vi "T7 Stream Error Handler KAG.vi"(8 "error in":errorcluster, 9 "Status Code":i32 format="%0.0f", 10 "Error Code":i32 format="%0.0f", 11 "Error Source":string) -> (0 "error out":errorcluster)   [LabVIEW 2022 SP3]
uses:
  <vilib>/Utility/error.llb/DialogType.ctl
panel:
  in  "Status Codes & Descriptions":cluster{"Codes":i32, "Descriptions":string}[](array[cluster])=[{"Codes"=2940, "Descriptions"="Auto-Recovery Active"}, {"Codes"=2941, "Descriptions"="Auto-Recovery End. Additional Status info = # scans skipped"}, {"Codes"=2942, "Descriptions"="Scan Overlap"}, {"Codes"=2943, "Descriptions"="Auto-Recovery End Overflow"}, {"Codes"=2944, "Descriptions"="Stream Burst Complete"}]
  in  "User-Defined Codes & Descriptions":cluster{"Codes":i32, "Descriptions":string}[](array[cluster])=[{"Codes"=6000, "Descriptions"="Empty Byte Array"}, {"Codes"=6001, "Descriptions"="Checksum Bad"}, {"Codes"=6002, "Descriptions"="Status Code"}, {"Codes"=6003, "Descriptions"="Transaction ID = NaN"}, {"Codes"=6004, "Descriptions"="Backlog Overflow"}]
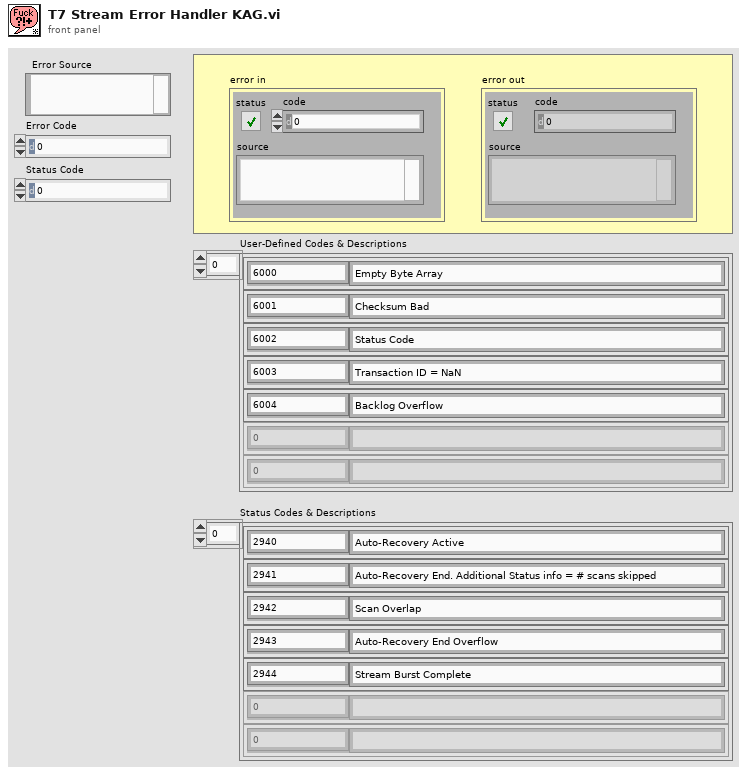
[diagram p1: front panel]
types:
  T1 = typedef "DialogType.ctl" = u16
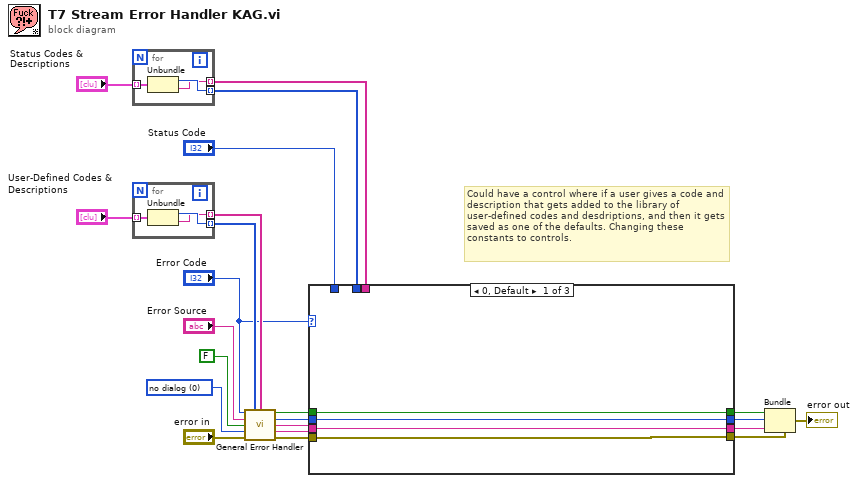
[diagram p0: block diagram]
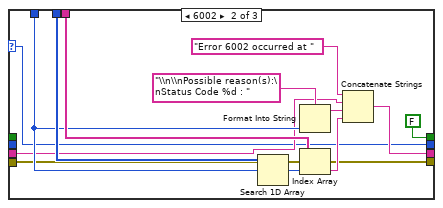
[diagram p2: hidden frame]
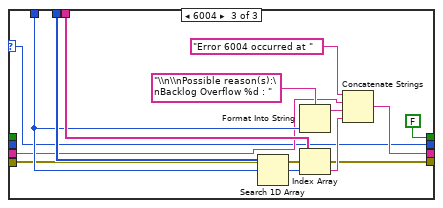
[diagram p3: hidden frame]
diagram:
  w22 = T1 0 items=["no dialog", "OK message", "continue or stop message", "OK message + warnings", "continue/stop + warnings"] ("type of dialog (OK msg:1)")
  # "Could have a control where if a user gives a code and description that gets added to the library of user-defined codes and desdriptions, and then it gets saved as one of the defaults. Changing these constants to controls."
  n1 = for {
    tunnel: "Status Codes & Descriptions" -> [w25] mode=indexing
    tunnel: [w24] -> w3 mode=indexing
    tunnel: [w23] -> w2 mode=indexing
    n2 = Unbundle(w25) -> ("Codes"=w24:i32, "Descriptions"=w23:string)
  }
  n3 = for {
    tunnel: "User-Defined Codes & Descriptions" -> [w28] mode=indexing
    tunnel: [w27] -> w17 mode=indexing
    tunnel: [w26] -> w16 mode=indexing
    n4 = Unbundle(w28) -> ("Codes"=w27:i32, "Descriptions"=w26:string)
  }
  n5 = call <vilib>:"General Error Handler.vi"("[error code] (0)"="Error Code", "[user-defined codes]"=w17, "[user-defined descriptions]"=w16, "[error source] (\" \")"="Error Source", "search ni.com link visible?(T)"=FALSE, "type of dialog (OK msg:1)"=w22, "error in (no error)"="error in") -> ("error?"=w12:bool, "code out"=w9:i32, "source out"=w1:string, "message"=w11:string, "error out"=w10:errorcluster)  [unwired: 4 in]
  n6 = case shown="0, Default" "Error Code" {
    selector: "Error Code" -> [_ w34 w47]
    tunnel: w12 -> [w32 _ _]
    tunnel: w11 -> [w30 _ _]
    tunnel: w10 -> [w29 w33 w46]
    tunnel: w9 -> [w31 _ _]
    tunnel: [w32 FALSE ("error?") FALSE ("error?")] -> w8
    tunnel: [w31 w34 w47] -> w7
    tunnel: [w30 w36 w49] -> w6
    tunnel: [w29 w33 w46] -> w5
    tunnel: "Status Code" -> [_ w42 w55]
    tunnel: w3 -> [_ w45 w58]
    tunnel: w2 -> [_ w43 w56]
    tunnel: w1 -> [_ w39 w52]
    frame 0, Default {
    }
    frame 6002 {
      n7 = Search 1D Array(1D array=w45, element=w42) -> (index of element=w44:i32)  [unwired: 1 in]
      n8 = Format Into String(format string="\\n\\nPossible reason(s):\nStatus Code %d : ", w42) -> (resulting string=w38:string)  [unwired: 2 in, 1 out]
      n9 = Index Array(array=w43, index=w44) -> (element=w37:string)
      n10 = Concatenate Strings("Error 6002 occurred at ", w39, w38, w37) -> (w36:string)
    }
    frame 6004 {
      n11 = Search 1D Array(1D array=w58, element=w55) -> (index of element=w57:i32)  [unwired: 1 in]
      n12 = Format Into String(format string="\\n\\nPossible reason(s):\nBacklog Overflow %d : ", w55) -> (resulting string=w51:string)  [unwired: 2 in, 1 out]
      n13 = Index Array(array=w56, index=w57) -> (element=w50:string)
      n14 = Concatenate Strings("Error 6004 occurred at ", w52, w51, w50) -> (w49:string)
    }
  }
  n15 = Bundle(cluster=w5, "status"=w8, "code"=w7, "source"=w6) -> (→"error out":errorcluster)
